vi "MHX Equivalent Diameter.vi"(10 "MHX Tube Diameter (m)":dbl, 11 "MHX Tube Pitch (m)":dbl) -> (3 "Numeric":dbl)   [LabVIEW 2019]
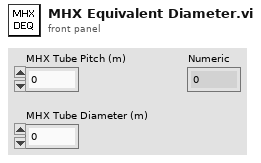
[diagram p1: front panel]
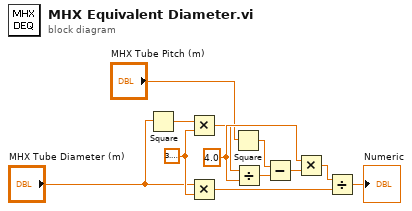
[diagram p0: block diagram]
diagram:
  w7 = 4.0 ("y")
  w9 = 3.141592653589793
  n1 = Square(x="MHX Tube Diameter (m)") -> (x^2=w3:dbl)
  n2 = Multiply(x=w3, y=w9) -> (x*y=w4:dbl)
  n3 = Multiply(x="MHX Tube Diameter (m)", y=w9) -> (x*y=w11:dbl)
  n4 = Square(x="MHX Tube Pitch (m)") -> (x^2=w2:dbl)
  n5 = Divide(x=w4, y=w7) -> (x/y=w5:dbl)
  n6 = Subtract(x=w2, y=w5) -> (x-y=w6:dbl)
  n7 = Multiply(x=w7, y=w6) -> (x*y=w10:dbl)
  n8 = Divide(x=w10, y=w11) -> (x/y=→"Numeric":dbl)
